vi "bnomoveX.vi"(8 "error in (no error)":errorcluster, 11 "X":dbl) -> (0 "error out":errorcluster)   [LabVIEW 2019]
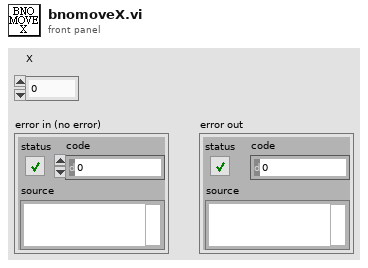
[diagram p1: front panel]
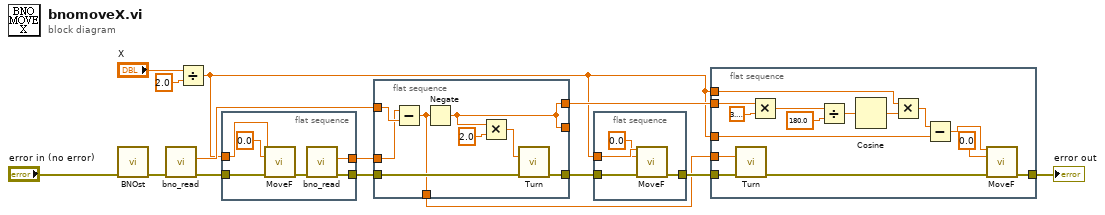
[diagram p0: block diagram]
diagram:
  n1 = call "BNOst.vi"("error in (no error)"="error in (no error)") -> ("error out"=w6:errorcluster)  [unwired: 10 in]
  n2 = call "bno_read.vi"("error in (no error)"=w6) -> ("error out"=w7:errorcluster, "x/y"=w8:dbl)  [unwired: 8 in]
  n3 = Divide(x="X", y=2.0) -> (x/y=w2:dbl)
  n4 = flat-sequence {
    tunnel: w7 -> [w20]
    tunnel: w2 -> [w15]
    tunnel: [w18] -> w13
    tunnel: [w17] -> w14
    frame #0 {
      n5 = call "MoveF.vi"("X"=w15, "Y"=0.0 ("X"), "error in (no error)"=w20) -> ("error out"=w19:errorcluster)  [unwired: 12 in]
      n6 = call "bno_read.vi"("error in (no error)"=w19) -> ("error out"=w18:errorcluster, "x/y"=w17:dbl)  [unwired: 8 in]
    }
  }
  n7 = flat-sequence {
    tunnel: w8 -> [w28]
    tunnel: [w22] -> w11
    tunnel: [w27] -> w3
    tunnel: w13 -> [w26]
    tunnel: w14 -> [w25]
    tunnel: [w22] -> _
    tunnel: [w21] -> w1
    frame #0 {
      n8 = Subtract(x=w25, y=w28) -> (x-y=w21:dbl)
      n9 = Negate(x=w21) -> (-x=w22:dbl)
      n10 = Multiply(x=w22, y=2.0) -> (x*y=w23:dbl)
      n11 = call "Turn.vi"("¨¤«×"=w23, "error in (no error)"=w26) -> ("error out"=w27:errorcluster)  [unwired: 13 in]
    }
  }
  n12 = flat-sequence {
    tunnel: [w32] -> w4
    tunnel: w3 -> [w31]
    tunnel: w2 -> [w30]
    frame #0 {
      n13 = call "MoveF.vi"("X"=w30, "Y"=0.0 ("X"), "error in (no error)"=w31) -> ("error out"=w32:errorcluster)  [unwired: 12 in]
    }
  }
  n14 = flat-sequence {
    tunnel: w2 -> [w47]
    tunnel: w11 -> [w45]
    tunnel: [w40] -> w12
    tunnel: w2 -> [w36]
    tunnel: w4 -> [w38]
    tunnel: w1 -> [w33]
    frame #0 {
      n15 = call "Turn.vi"("¨¤«×"=w33, "error in (no error)"=w38) -> ("error out"=w39:errorcluster)  [unwired: 13 in]
      n16 = Multiply(x=w45, y=3.141592653589793) -> (x*y=w42:dbl)
      n17 = Divide(x=w42, y=180.0) -> (x/y=w41:dbl)
      n18 = Cosine(x=w41) -> (cos(x)=w46:dbl)
      n19 = Multiply(x=w47, y=w46) -> (x*y=w37:dbl)
      n20 = Subtract(x=w37, y=w36) -> (x-y=w35:dbl)
      n21 = call "MoveF.vi"("X"=w35, "Y"=0.0 ("X"), "error in (no error)"=w39) -> ("error out"=w40:errorcluster)  [unwired: 12 in]
    }
  }
  "error out" <- w12
